vi "database_path.vi"() -> (2 "database path":path)   [LabVIEW 2018]
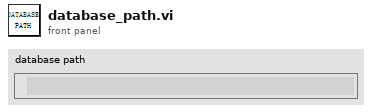
[diagram p1: front panel]
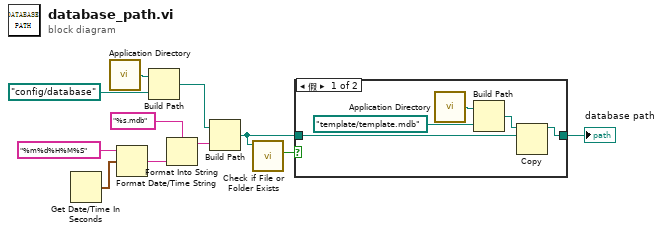
[diagram p0: block diagram]
diagram:
  n1 = Get Date/Time In Seconds() -> (seconds since 1Jan1904=w3:timestamp)
  n2 = call <vilib>:"Application Directory.vi"() -> ("Application Directory"=w10:path)
  n3 = Format Date/Time String(time format string (%c)="%m%d%H%M%S" ("时间格式字符串(%c)"), seconds (now)=w3) -> (date/time string=w1:string)  [unwired: 1 in]
  n4 = Build Path(base path=w10, name or relative path=path "config/database" ("Application Directory")) -> (appended path=w8:path)
  n5 = Format Into String(format string="%s.mdb" ("格式字符串"), w1) -> (resulting string=w7:string)  [unwired: 2 in, 1 out]
  n6 = Build Path(base path=w8, name or relative path=w7) -> (appended path=w5:path)
  n7 = call <vilib>:"Check if File or Folder Exists.vi"("path"=w5) -> ("file or folder exists?"=w4:bool)  [unwired: 8 in, 2 out]
  n8 = case shown="假" w4 {
    tunnel: [w16 w17] -> w6
    tunnel: w5 -> [w15 w17]
    frame False {
      n9 = call <vilib>:"Application Directory.vi"() -> ("Application Directory"=w14:path)
      n10 = Build Path(base path=w14, name or relative path=path "template/template.mdb" ("Application Directory")) -> (appended path=w12:path)
      n11 = Copy(10:w15, 11:w12) -> (3:w16:path)  [unwired: 3 in, 2 out]
    }
    frame True {
    }
  }
  "database path" <- w6
